vi "TAT_Planner_creator.vi"(8 "error in (no error)":errorcluster) -> (0 "error out":errorcluster)   [LabVIEW 2017]
uses:
  <vilib>/addons/database/Connection.llb/Conn ObjectReference.ctl
  b1939813-2d0c-4b6e-8ee7-2e1edd5edc28.vi
  <vilib>/Utility/config.llb/Read Key (I32).vi
  <vilib>/Utility/config.llb/Read Key (String).vi
  <userlib>/_OpenG.lib/array/array.llb/Remove Duplicates from 1D Array (String)__ogtk.vi
  <vilib>/Utility/config.llb/NI_LVConfig.lvlib
  <vilib>/addons/database/NI_Database_API.lvlib
panel:
  in  "BOX CALCULATION":bool
  out "PART LIST 6":string(tree)
  out "PART LIST 5":string(tree)
  out "PART LIST 4":string(tree)
  out "PART LIST 3":string(tree)
  out "PART LIST 2":string(tree)
  out "PART LIST 1":string(tree)
  out "PLANNED TABLE":string[][](table)
  in  "QTY 6":u32
  in  "TABLE DRAWING 6":string(combo)
  in  "COLOR 6":string(combo)
  in  "QTY 5":u32
  in  "TABLE DRAWING 5":string(combo)
  in  "COLOR 5":string(combo)
  in  "QTY 4":u32
  in  "TABLE DRAWING 4":string(combo)
  in  "COLOR 4":string(combo)
  in  "QTY 3":u32
  in  "TABLE DRAWING 3":string(combo)
  in  "COLOR 3":string(combo)
  in  "QTY 2":u32
  in  "TABLE DRAWING 2":string(combo)
  in  "COLOR 2":string(combo)
  in  "QTY 1":u32
  out "Array 2":string[][](array[string])
  out "Array":string[][](array[string])
  in  "TABLE DRAWING 1":string(combo)
  in  "WORK ORDER":string
  in  "COUNTRY":string(combo)
  in  "COLOR 1":string(combo)
  in  "MODEL":string(combo)
  in  "PLAN DATE":timestamp format="%<%x>T"
  in  "Cancle":bool
  in  "EDIT & SAVE":bool
  in  "CHILD PART CLUSTER":T1
  in  "CANCLE 3":bool
  in  "PRINTING":bool
  in  "Manual print":bool
  in  "Cancle 2":bool
  in  "Delete Button":bool
  in  "HOME":bool
  in  "UPDATE TABLE":bool
  in  "Tab Control":enum32{"Child Part Creator", "Varient Adding"}(tab)
  in  "CHILD PART NAME":string(combo)
  in  "Save Button":bool
  in  "QTY PER BOX":i32=1 min=1 max=100 step=1
  in  "Delete Square":bool
  in  "BOX WEIGHT":u16=1 min=1 max=100 step=1 format="%.0f gm"
  in  "BOX RH PART QUANTITY":u16=1 min=1 max=100 step=1
  in  "PART NUMBER":u16=1 min=1 max=100 step=1
  out "Varient Details":string[][](table)
  # "Export Plan Creator"
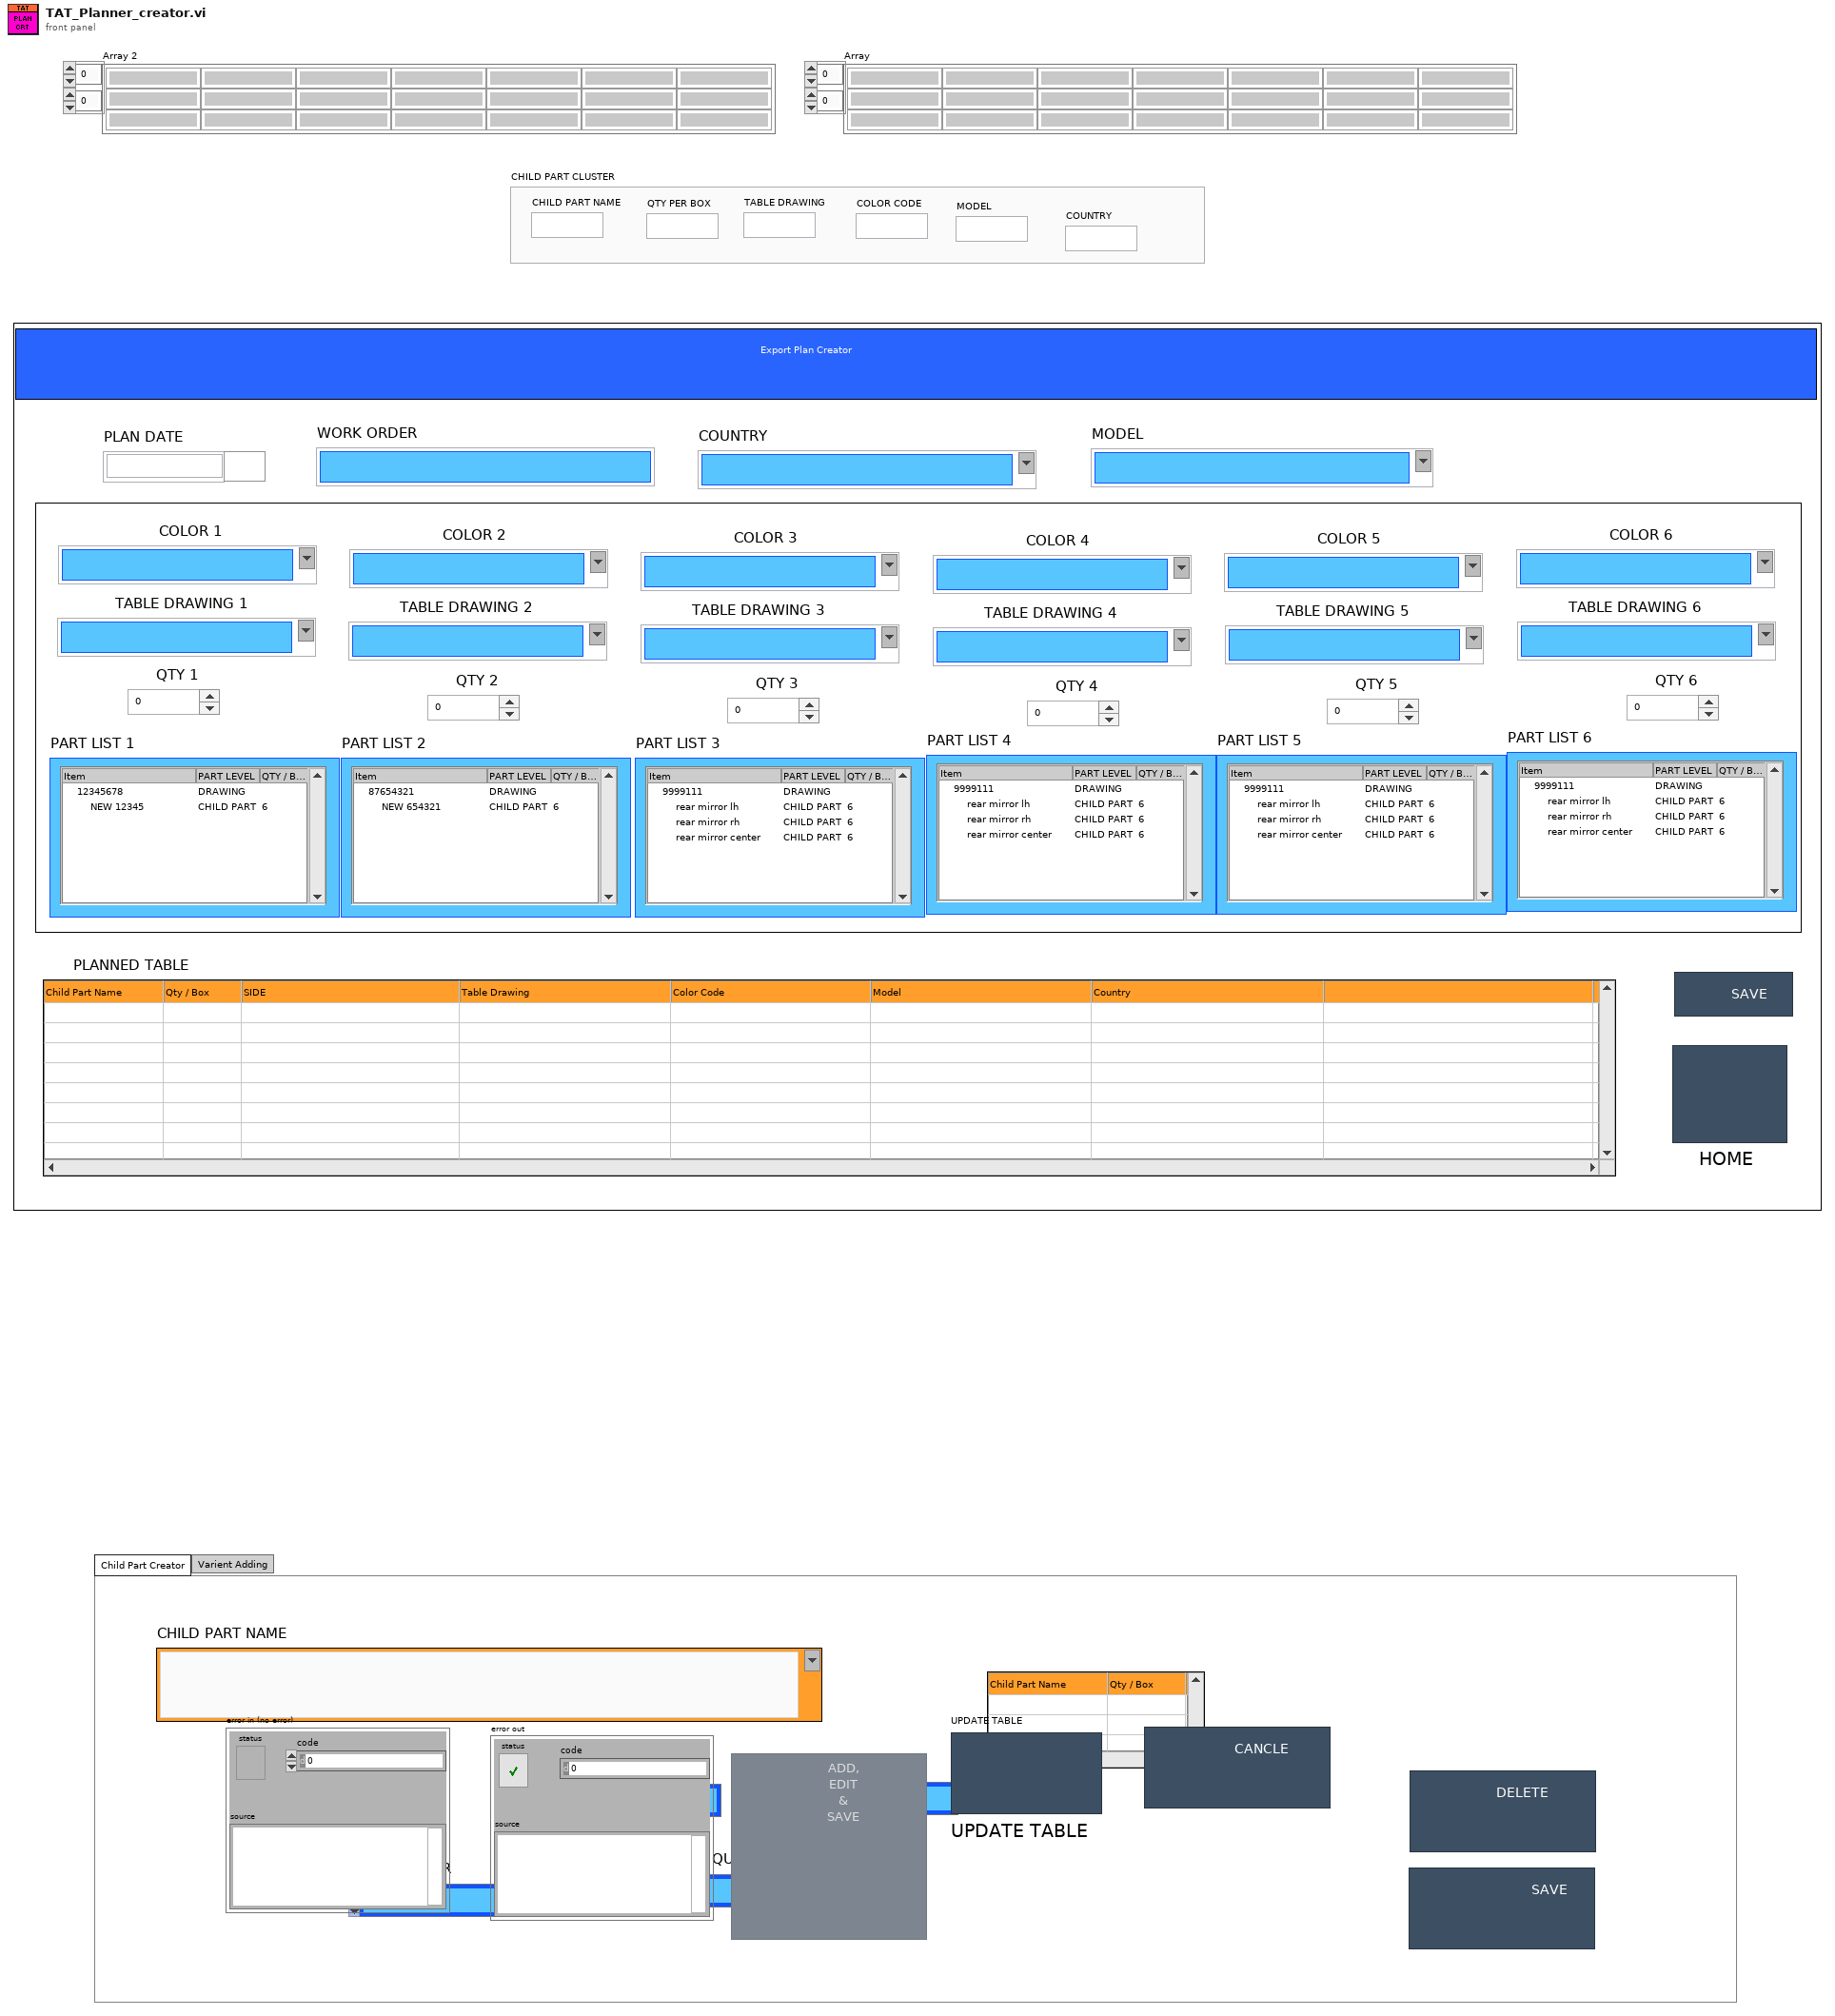
[diagram p1: front panel]
types:
  T1 = cluster{"CHILD PART NAME":string, "QTY PER BOX":string, "TABLE DRAWING":string, "COLOR CODE":string, "MODEL":string, "COUNTRY":string}
  T2 = enum32{"invalid app kind", "Development System", "Run Time System", "Student Edition", "Embedded LabVIEW", "Evaluation", "Custom"}
  T3 = typedef "NI_Database_API.lvlib/Conn ObjectReference.ctl" = refnum<k1>
  T4 = cluster{"Varient number":u16, "Part name":string, "connection reference":T3, "Batch_Size":u16, "PART_NO":string, "TORISHI_CODE":string, "scanner com":refnum<visa-resource-name>, "Part Name List":string[], "Varient path":path, "Current Varient path":path, "Communication path":path, "Package path":path, "Part PRN path":path, "Station2 printer IP":string, "Station1 printer IP":string, "Current Serial Number":string, "Station1_QR":string, "Serial_Number":path, "PRIVIOUS code":string[], "Barcode station2 log":string, "Barcode station2 Up":string, "HARNESS CODE":string, "Station 1 bypass":bool}
  T5 = cluster{"COLOR":string[], "MODEL":string[], "TABLE DRAWING":string[], "COUNTRY":string[]}
  T6 = typedef "NI_LVConfig.lvlib/Config Data RefNum.ctl" = refnum<k1>
  T7 = cluster{"QTY PER BOX":i32, "TABLE DRAWING":string, "COLOR CODE":string, "MODEL":string, "COUNTRY":string}
  T8 = enum8{"Enabled", "Disabled", "Disabled and Grayed Out"}
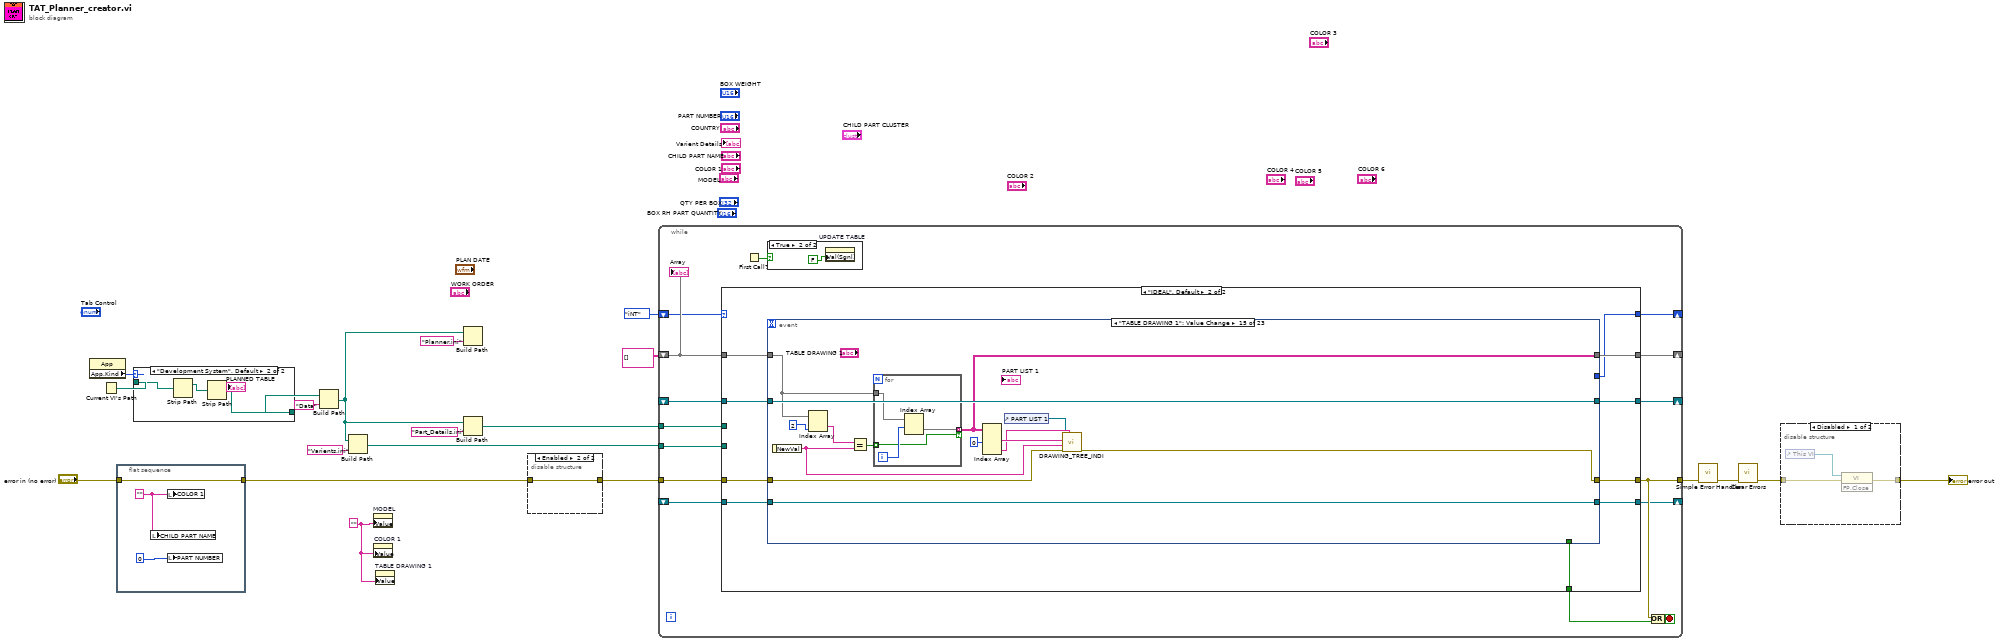
[diagram p0: block diagram]
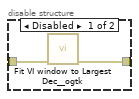
[diagram p2: hidden frame]
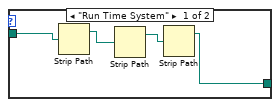
[diagram p4: hidden frame]
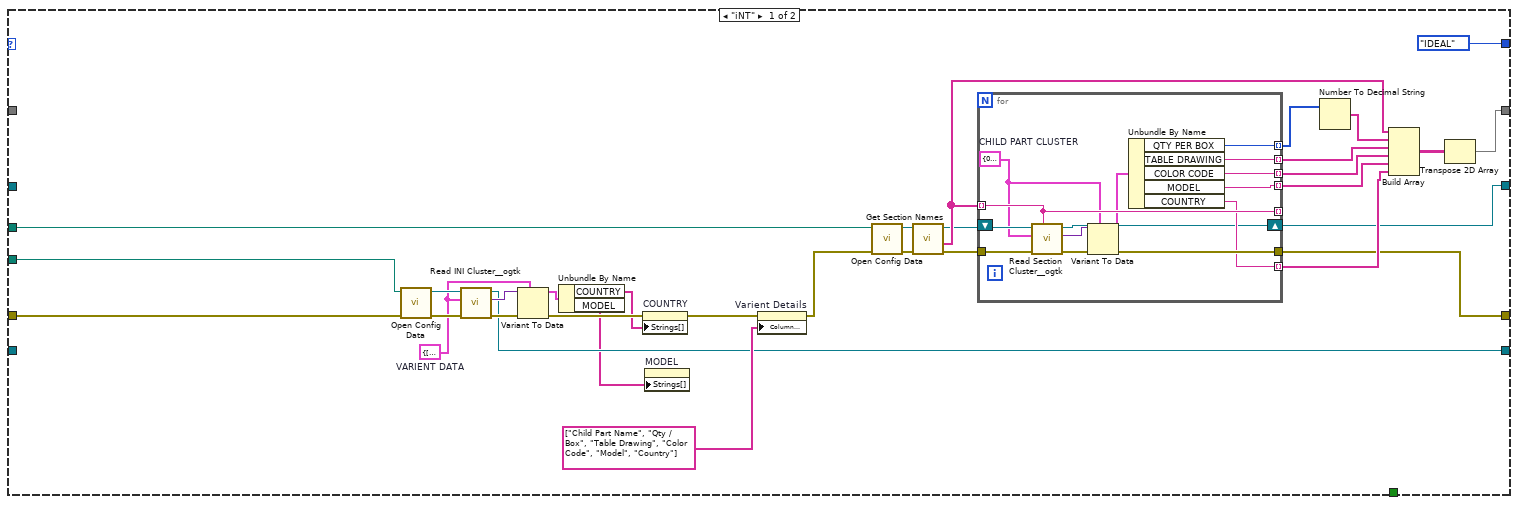
[diagram p5: hidden frame]
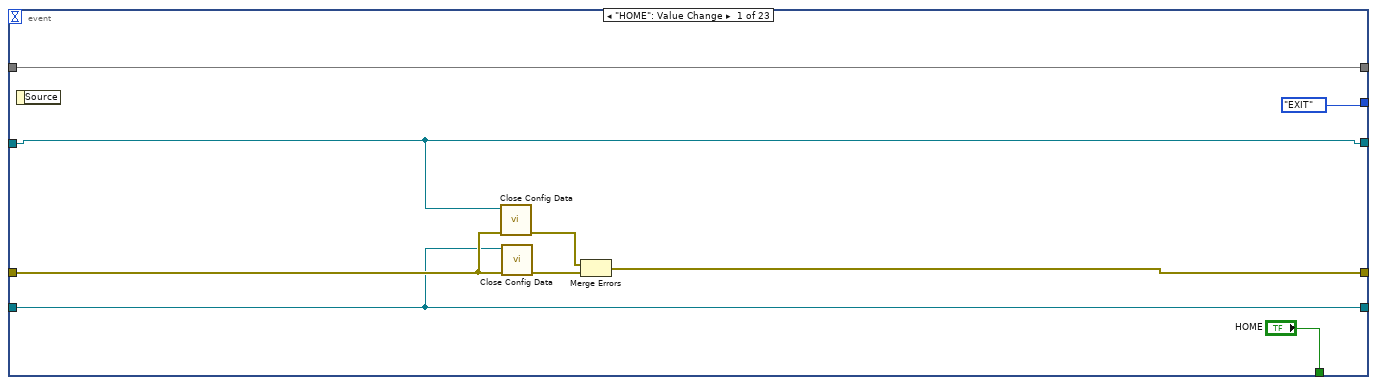
[diagram p6: hidden frame]
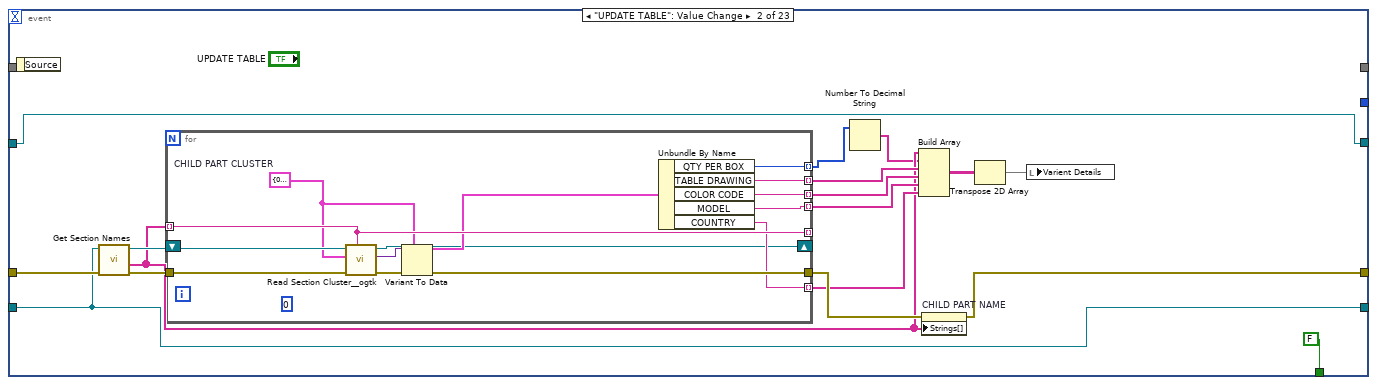
[diagram p7: hidden frame]
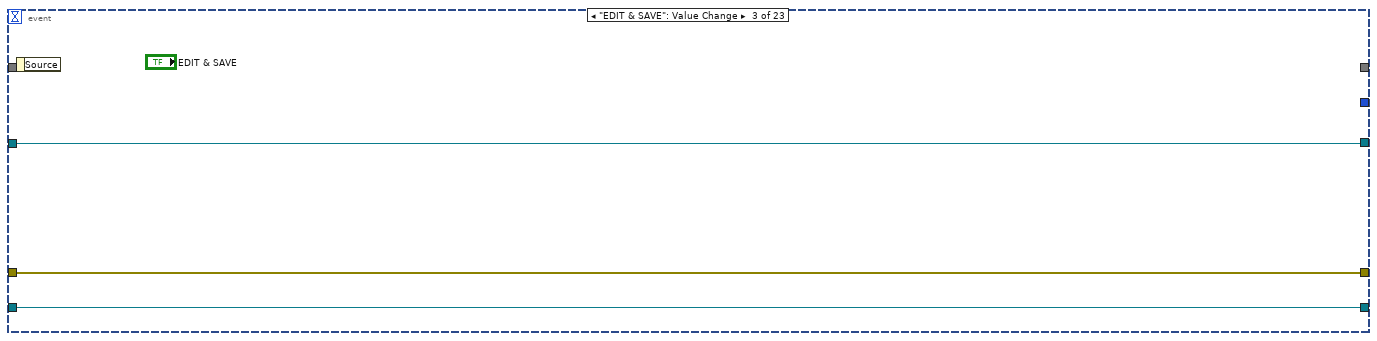
[diagram p8: hidden frame]
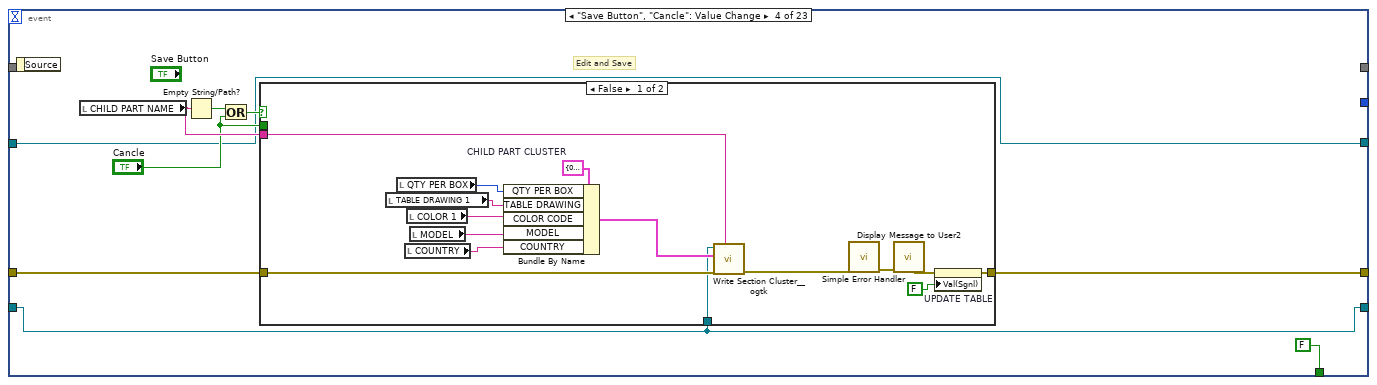
[diagram p9: hidden frame]
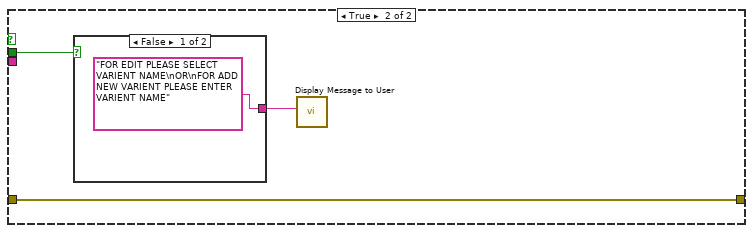
[diagram p10: hidden frame]
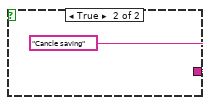
[diagram p11: hidden frame]
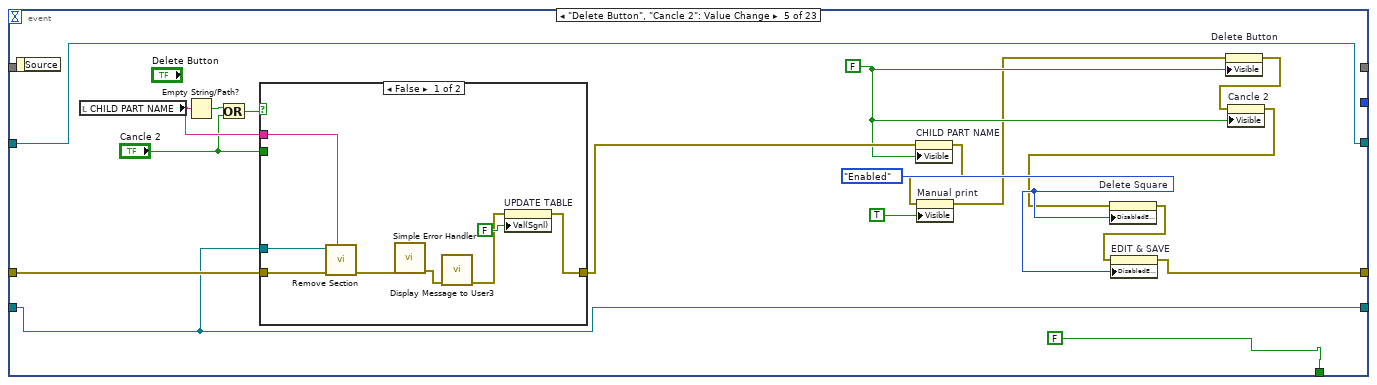
[diagram p12: hidden frame]
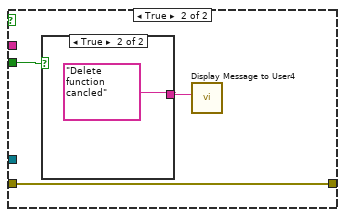
[diagram p13: hidden frame]
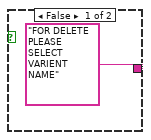
[diagram p14: hidden frame]
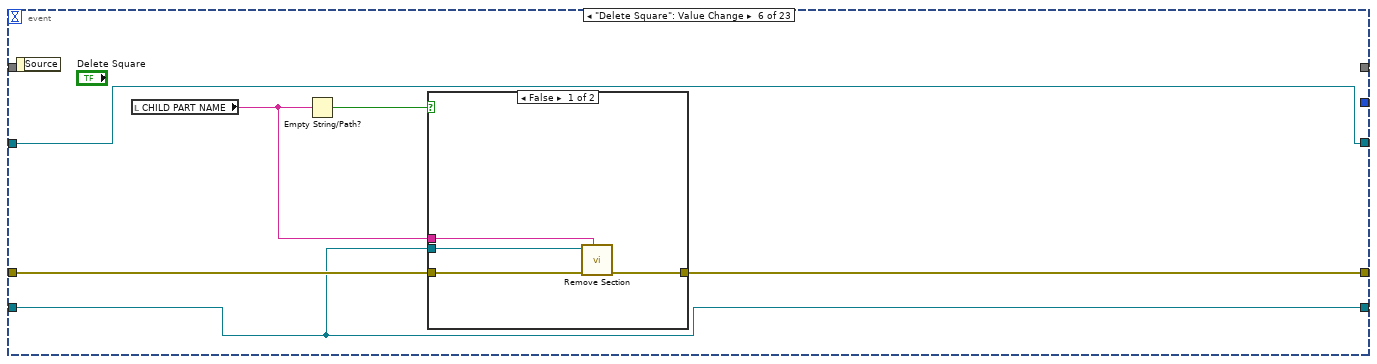
[diagram p15: hidden frame]
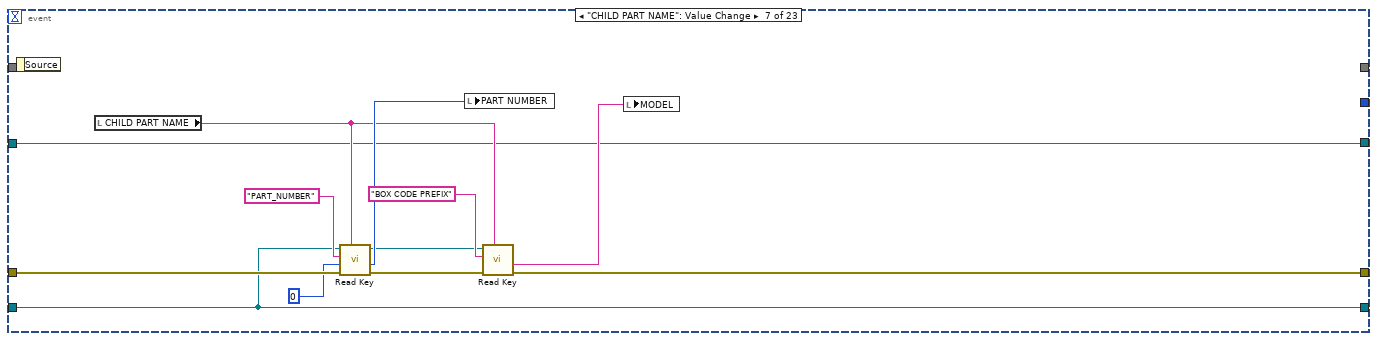
[diagram p17: hidden frame]
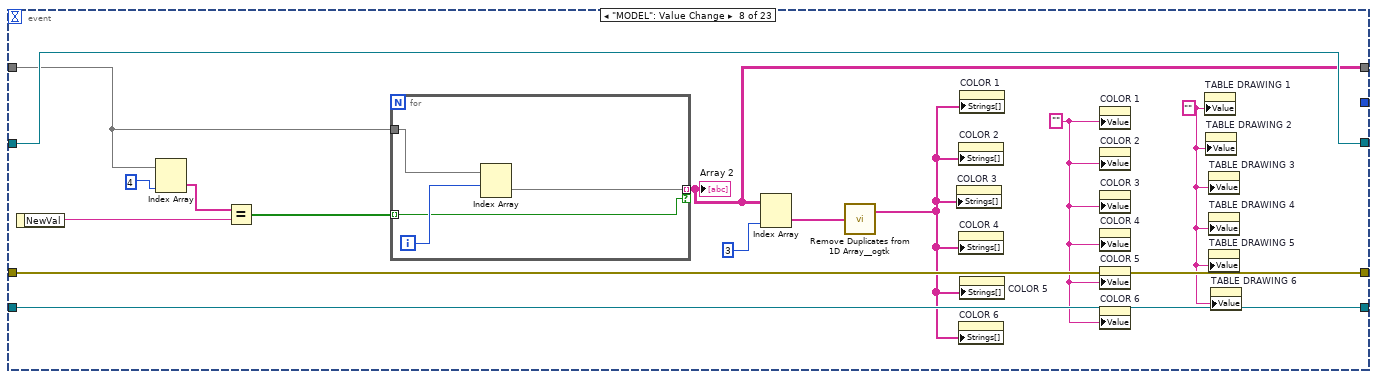
[diagram p18: hidden frame]
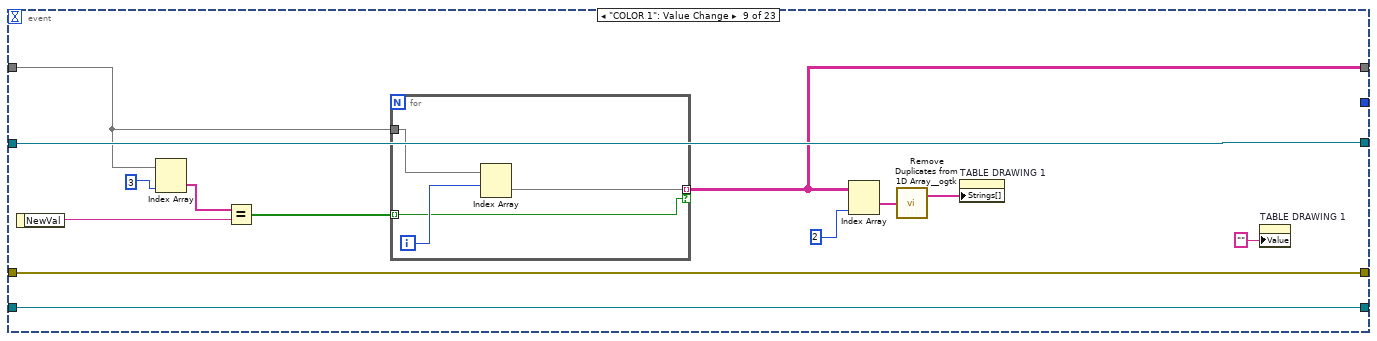
[diagram p19: hidden frame]
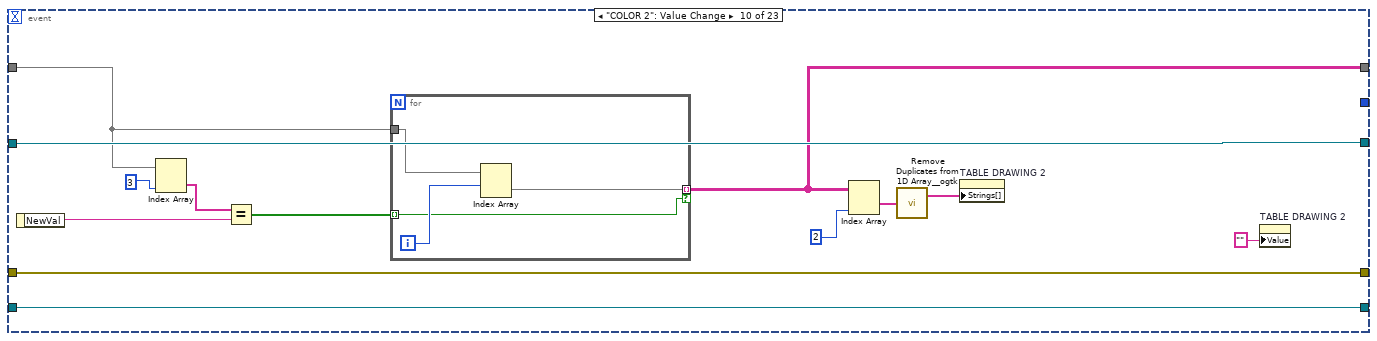
[diagram p20: hidden frame]
diagram:
  w4 = ""
  n1 = property class="App"() -> ("App.Kind"=w15:T2)  [unwired: 2 in, 2 out]
  n2 = Current VI's Path() -> (path=w16:path)
  n3 = flat-sequence {
    tunnel: [w21] -> w11
    tunnel: "error in (no error)" -> [w21]
    frame #0 {
      w23 = "" ("PART NUMBER")
      n4 = local write "CHILD PART NAME"(w23) -> ()
      n5 = local write "COLOR 1"(w23) -> ()
      n6 = local write "PART NUMBER"(u16 0 ("BATCH SIZE")) -> ()
    }
  }
  n7 = case shown="\"Development System\", Default" w15 {
    tunnel: w16 -> [w25 w29]
    tunnel: [w24 w28] -> w9
    frame "Run Time System" {
      n8 = Strip Path(path=w25) -> (stripped path=w27:path)  [unwired: 1 out]
      n9 = Strip Path(path=w27) -> (stripped path=w26:path)  [unwired: 1 out]
      n10 = Strip Path(path=w26) -> (stripped path=w24:path)  [unwired: 1 out]
    }
    frame "Development System", Default {
      n11 = Strip Path(path=w29) -> (stripped path=w30:path)  [unwired: 1 out]
      n12 = Strip Path(path=w30) -> (stripped path=w28:path)  [unwired: 1 out]
    }
  }
  n13 = Build Path(base path=w9, name or relative path="Data") -> (appended path=w6:path)
  n14 = Build Path(base path=w6, name or relative path="Varients.ini") -> (appended path=w2:path)
  n15 = property on="MODEL" class="CmbBox"("Value"=w4) -> ()  [unwired: 2 in, 2 out]
  n16 = property on="COLOR 1" class="CmbBox"("Value"=w4) -> ()  [unwired: 2 in, 2 out]
  n17 = property on="TABLE DRAWING 1" class="CmbBox"("Value"=w4) -> ()  [unwired: 2 in, 2 out]
  n18 = Build Path(base path=w6, name or relative path="Planner.ini") -> ()  [unwired: 1 out]
  n19 = Build Path(base path=w6, name or relative path="Part_Details.ini") -> (appended path=w7:path)
  n20 = disable-structure shown="Enabled" {
    disable-tunnel: w11 -> [w32 w33]
    disable-tunnel: [w31 w33] -> w8
    frame Disabled {
      n21 = call <userlib>:"Fit VI window to Largest Dec__ogtk.vi"("error in (no error)"=w32) -> ("error out"=w31:errorcluster)  [unwired: 5 in, 1 out]
    }
    frame Enabled {
    }
  }
  n22 = while {
    tunnel: w8 -> [w47]
    tunnel: [w45] -> w17
    tunnel: w7 -> [w40]
    shift-right: [w43] -> _
    shift-left: string[][] [] -> [w42]
    shift-right: [w34] -> _
    shift-left: enum16{"iNT", "IDEAL", "EXIT"}."iNT" -> [w41]
    shift-right: [w39] -> _
    shift-left: _ -> [w38]
    tunnel: w2 -> [w37]
    shift-right: [w36] -> _
    shift-left: _ -> [w35]
    stop <- w46 stop-if-true
    n23 = case shown="\"IDEAL\", Default" w41 {
      tunnel: [_ w104] -> w48
      tunnel: w47 -> [w54 w103]
      tunnel: [w70 w102] -> w45
      tunnel: [w65 w101] -> w43
      tunnel: w42 -> [_ w100]
      tunnel: w40 -> [w68 _]
      tunnel: [w66 w98] -> w39
      tunnel: w38 -> [_ w99]
      tunnel: w37 -> [w52 _]
      tunnel: [w51 w96] -> w36
      tunnel: w35 -> [_ w97]
      tunnel: [enum16{"iNT", "IDEAL", "EXIT"}."IDEAL" w95] -> w34
      frame "iNT" {
        w56 = T5 {"COLOR"=[], "MODEL"=[], "TABLE DRAWING"=[], "COUNTRY"=[]}  # VARIENT DATA
        n24 = call <vilib>:"Open Config Data.vi"("error in (no error)"=w54, "configuration file path"=w52) -> ("error out"=w62:errorcluster, "refnum"=w63:T6)  [unwired: 7 in, 1 out]
        n25 = call <userlib>:"Read INI Cluster__ogtk.vi"("error in (no error)"=w62, "INI Fomatted Cluster Type"=w56, "refnum"=w63) -> ("error out"=w61:errorcluster, "INI Fomatted Cluster"=w64:variant, "dup refnum"=w51:T6)  [unwired: 4 in, 2 out]
        n26 = Variant To Data(error in=w61, type=w56, Variant=w64) -> (data=w58:T5, error out=w60:errorcluster)
        n27 = Unbundle By Name(w58) -> ("COUNTRY"=w57:string[], "MODEL"=w49:string[])
        n28 = property on="COUNTRY" class="CmbBox"(error in=w60, "Strings[]"=w57) -> (error out=w59:errorcluster)  [unwired: 1 in, 1 out]
        n29 = property on="MODEL" class="CmbBox"("Strings[]"=w49) -> ()  [unwired: 2 in, 2 out]
        n30 = property on="Varient Details" class="Tbl (strict)"(error in=w59, "Column Headers[]"=string[] ["Child Part Name", "Qty / Box", "Table Drawing", "Color Code", "Model", "Country"] ("Column Header Strings[]")) -> (error out=w53:errorcluster)  [unwired: 1 in, 1 out]
        n31 = call <vilib>:"Open Config Data.vi"("error in (no error)"=w53, "configuration file path"=w68) -> ("error out"=w69:errorcluster, "refnum"=w67:T6)  [unwired: 7 in, 1 out]
        n32 = call <vilib>:"Get Section Names.vi"("error in (no error)"=w69, "refnum"=w67) -> ("error out"=w72:errorcluster, "section names"=w78:string[], "refnum out"=w73:T6)  [unwired: 7 in]
        n33 = for {
          tunnel: [w90] -> w70
          tunnel: w72 -> [w94]
          tunnel: w78 -> [w92] mode=indexing
          tunnel: [w92] -> _ mode=indexing
          tunnel: [w87] -> w79 mode=indexing
          tunnel: [w86] -> w74 mode=indexing
          tunnel: [w85] -> w75 mode=indexing
          tunnel: [w84] -> w76 mode=indexing
          tunnel: [w83] -> w77 mode=indexing
          shift-right: [w82] -> w66
          shift-left: w73 -> [w93]
          w81 = T7 {"QTY PER BOX"=0, "TABLE DRAWING"="", "COLOR CODE"="", "MODEL"="", "COUNTRY"=""}  # CHILD PART CLUSTER
          n34 = call <userlib>:"Read Section Cluster__ogtk.vi"("section (optional)"=w92, "error in (no error)"=w94, "Section Formatted Cluster Type"=w81, "refnum"=w93) -> ("error out"=w91:errorcluster, "Section Formatted Cluster"=w89:variant, "dup refnum"=w82:T6)  [unwired: 3 in, 2 out]
          n35 = Variant To Data(error in=w91, type=w81, Variant=w89) -> (data=w88:T7, error out=w90:errorcluster)
          n36 = Unbundle By Name(w88) -> ("QTY PER BOX"=w87:i32, "TABLE DRAWING"=w86:string, "COLOR CODE"=w85:string, "MODEL"=w84:string, "COUNTRY"=w83:string)
        }
        n37 = Number To Decimal String(number=w79) -> (decimal integer string=w80:string[])  [unwired: 1 in]
        n38 = Build Array(w78, w80, w74, w75, w76, w77) -> (w71:string[][])
        n39 = Transpose 2D Array(2D array=w71) -> (transposed array=w65:string[][])
      }
      frame "IDEAL", Default {
        n40 = event shown="[14] \"TABLE DRAWING 1\": Value Change" {
          selector: _ -> [_ _ _ _ _ _ _ _ _ _ _ _ _ _ _ _ _ _ _ _ _ _ _]
          dyn-events: _ -> [_ _ _ _ _ _ _ _ _ _ _ _ _ _ _ _ _ _ _ _ _ _ _]
          timeout: _ -> [_ _ _ _ _ _ _ _ _ _ _ _ _ _ _ _ _ _ _ _ _ _ _]
          tunnel: ["HOME" FALSE ("stop") _ FALSE ("stop") FALSE ("stop") _ _ _ _ _ _ _ _ _ _ _ _ _ _ _ _ _ _] -> w104
          tunnel: w103 -> [w111 w120 w147 w155 w193 w213 w230 w244 w261 w278 w295 w312 w329 w346 w364 w373 w387 w405 w423 w441 w459 w468 w485]
          tunnel: [w106 w119 w147 w150 w185 w212 w223 w244 w261 w278 w295 w312 w329 w346 w352 w373 w375 w393 w411 w429 w447 w467 w475] -> w102
          tunnel: [w110 _ _ _ _ _ _ w235 w251 w268 w285 w302 w319 w336 w357 w370 w380 w398 w416 w434 w452 _ _] -> w101
          tunnel: w100 -> [w110 _ _ _ _ _ _ w236 w252 w269 w286 w303 w320 w337 w358 w370 w381 w399 w417 w435 w453 _ _]
          tunnel: w99 -> [w109 w115 w146 w149 w178 w209 w220 w243 w259 w276 w293 w310 w327 w344 w363 w372 w386 w404 w422 w440 w458 w465 w472]
          tunnel: [w109 w115 w146 w149 w178 w209 w220 w243 w259 w276 w293 w310 w327 w344 w363 w372 w386 w404 w422 w440 w458 w465 w472] -> w98
          tunnel: w97 -> [w108 w114 w145 w148 w177 w208 w219 w242 w258 w275 w292 w309 w326 w343 w362 w371 w385 w403 w421 w439 w457 w464 w471]
          tunnel: [w108 w114 w145 w148 w177 w208 w219 w242 w258 w275 w292 w309 w326 w343 w362 w371 w385 w403 w421 w439 w457 w464 w471] -> w96
          tunnel: [enum16{"iNT", "IDEAL", "EXIT"}."EXIT" _ _ _ _ _ _ _ _ _ _ _ _ _ _ _ _ _ _ _ _ _ _] -> w95
          event "HOME": Value Change {
            n41 = event-data() -> ()  [unwired: 1 in, 1 out]
            n42 = call <vilib>:"Close Config Data.vi"("error in (no error)"=w111, "refnum"=w109) -> ("error out"=w105:errorcluster)  [unwired: 8 in, 1 out]
            n43 = call <vilib>:"Close Config Data.vi"("error in (no error)"=w111, "refnum"=w108) -> ("error out"=w112:errorcluster)  [unwired: 8 in, 1 out]
            n44 = Merge Errors(w105, w112) -> (w106:errorcluster)
          }
          event "UPDATE TABLE": Value Change {
            n45 = event-data() -> ()  [unwired: 1 in, 1 out]
            n46 = call <vilib>:"Get Section Names.vi"("error in (no error)"=w120, "refnum"=w114) -> ("error out"=w128:errorcluster, "section names"=w118:string[], "refnum out"=w127:T6)  [unwired: 7 in]
            n47 = for {
              tunnel: [w140] -> w126
              tunnel: w128 -> [w144]
              tunnel: w118 -> [w142] mode=indexing
              tunnel: [w142] -> _ mode=indexing
              tunnel: [w137] -> w117 mode=indexing
              tunnel: [w136] -> w124 mode=indexing
              tunnel: [w135] -> w123 mode=indexing
              tunnel: [w134] -> w122 mode=indexing
              tunnel: [w133] -> w121 mode=indexing
              shift-right: [w132] -> _
              shift-left: w127 -> [w143]
              w131 = T7 {"QTY PER BOX"=0, "TABLE DRAWING"="", "COLOR CODE"="", "MODEL"="", "COUNTRY"=""}  # CHILD PART CLUSTER
              (unwired) 0 ("default value")
              n48 = call <userlib>:"Read Section Cluster__ogtk.vi"("section (optional)"=w142, "error in (no error)"=w144, "Section Formatted Cluster Type"=w131, "refnum"=w143) -> ("error out"=w141:errorcluster, "Section Formatted Cluster"=w139:variant, "dup refnum"=w132:T6)  [unwired: 3 in, 2 out]
              n49 = Variant To Data(error in=w141, type=w131, Variant=w139) -> (data=w138:T7, error out=w140:errorcluster)
              n50 = Unbundle By Name(w138) -> ("QTY PER BOX"=w137:i32, "TABLE DRAWING"=w136:string, "COLOR CODE"=w135:string, "MODEL"=w134:string, "COUNTRY"=w133:string)
            }
            n51 = Number To Decimal String(number=w117) -> (decimal integer string=w116:string[])  [unwired: 1 in]
            n52 = Build Array(w118, w116, w124, w123, w122, w121) -> (w129:string[][])
            n53 = property on="CHILD PART NAME" class="CmbBox"(error in=w126, "Strings[]"=w118) -> (error out=w119:errorcluster)  [unwired: 1 in, 1 out]
            n54 = Transpose 2D Array(2D array=w129) -> (transposed array=w125:string[][])
            n55 = local write "Varient Details"(w125) -> ()
          }
          event "EDIT & SAVE": Value Change {
            n56 = event-data() -> ()  [unwired: 1 in, 1 out]
          }
          event "Save Button", "Cancle": Value Change {
            # "Edit and Save"
            n57 = event-data() -> ()  [unwired: 1 in, 1 out]
            n58 = local read "CHILD PART NAME"() -> (w154:string)
            n59 = Empty String/Path?(string/path=w154) -> (empty?=w153:bool)
            n60 = Or(x=w153, y="Cancle") -> (x .or. y?=w152:bool)
            n61 = case shown="False" w152 {
              tunnel: w155 -> [w171 w174]
              tunnel: [w169 w174] -> w150
              tunnel: w154 -> [w165 _]
              tunnel: "Cancle" -> [_ w172]
              tunnel: w148 -> [w157 _]
              frame False {
                w159 = T7 {"QTY PER BOX"=0, "TABLE DRAWING"="", "COLOR CODE"="", "MODEL"="", "COUNTRY"=""}  # CHILD PART CLUSTER
                n62 = local read "TABLE DRAWING 1"() -> (w161:string)
                n63 = local read "QTY PER BOX"() -> (w160:i32)
                n64 = local read "COUNTRY"() -> (w164:string)
                n65 = local read "COLOR 1"() -> (w162:string)
                n66 = local read "MODEL"() -> (w163:string)
                n67 = Bundle By Name(cluster=w159, "QTY PER BOX"=w160, "TABLE DRAWING"=w161, "COLOR CODE"=w162, "MODEL"=w163, "COUNTRY"=w164) -> (w158:T7)
                n68 = call <userlib>:"Write Section Cluster__ogtk.vi"("section (optional)"=w165, "error in (no error)"=w171, "Section Formatted Cluster"=w158, "refnum"=w157) -> ("error out"=w166:errorcluster)  [unwired: 6 in, 1 out]
                n69 = call <vilib>:"Simple Error Handler.vi"("error in (no error)"=w166) -> ("error out"=w168:errorcluster)  [unwired: 4 in, 4 out]
                n70 = call "Display Message to User2"("error in (no error)"=w168) -> ("error out"=w167:errorcluster)  [unwired: 9 in, 1 out]
                n71 = property on="UPDATE TABLE" class="Bool (strict)"(error in=w167, "Val(Sgnl)"=FALSE) -> (error out=w169:errorcluster)  [unwired: 1 in, 1 out]
              }
              frame True {
                n72 = case shown="False" w172 {
                  tunnel: ["FOR EDIT PLEASE SELECT VARIENT NAME\nOR\nFOR ADD NEW VARIENT PLEASE ENTER VARIENT NAME" "Cancle saving"] -> w173
                  frame False {
                  }
                  frame True {
                  }
                }
                n73 = call "Display Message to User"("Message"=w173) -> ()  [unwired: 9 in, 2 out]
              }
            }
          }
          event "Delete Button", "Cancle 2": Value Change {
            w187 = T8."Enabled" ("Disabled")
            w182 = FALSE
            n74 = event-data() -> ()  [unwired: 1 in, 1 out]
            n75 = local read "CHILD PART NAME"() -> (w192:string)
            n76 = Empty String/Path?(string/path=w192) -> (empty?=w191:bool)
            n77 = Or(x=w191, y="Cancle 2") -> (x .or. y?=w190:bool)
            n78 = case shown="False" w190 {
              tunnel: w193 -> [w197 w205]
              tunnel: [w201 w205] -> w186
              tunnel: w192 -> [w198 _]
              tunnel: "Cancle 2" -> [_ w204]
              tunnel: w177 -> [w195 _]
              frame False {
                n79 = call <vilib>:"Remove Section.vi"("section"=w198, "error in (no error)"=w197, "refnum"=w195) -> ("error out"=w196:errorcluster)  [unwired: 6 in, 2 out]
                n80 = call <vilib>:"Simple Error Handler.vi"("error in (no error)"=w196) -> ("error out"=w200:errorcluster)  [unwired: 4 in, 4 out]
                n81 = call "Display Message to User3"("error in (no error)"=w200) -> ("error out"=w199:errorcluster)  [unwired: 9 in, 1 out]
                n82 = property on="UPDATE TABLE" class="Bool (strict)"(error in=w199, "Val(Sgnl)"=FALSE) -> (error out=w201:errorcluster)  [unwired: 1 in, 1 out]
              }
              frame True {
                n83 = case shown="True" w204 {
                  tunnel: ["FOR DELETE PLEASE SELECT VARIENT NAME" "Delete function cancled"] -> w203
                  frame False {
                  }
                  frame True {
                  }
                }
                n84 = call "Display Message to User4"("Message"=w203) -> ()  [unwired: 9 in, 2 out]
              }
            }
            n85 = property on="CHILD PART NAME" class="CmbBox"(error in=w186, "Visible"=w182) -> (error out=w180:errorcluster)  [unwired: 1 in, 1 out]
            n86 = property on="Manual print" class="Bool"(error in=w180, "Visible"=TRUE) -> (error out=w179:errorcluster)  [unwired: 1 in, 1 out]
            n87 = property on="Delete Button" class="Bool"(error in=w179, "Visible"=w182) -> (error out=w184:errorcluster)  [unwired: 1 in, 1 out]
            n88 = property on="Cancle 2" class="Bool"(error in=w184, "Visible"=w182) -> (error out=w183:errorcluster)  [unwired: 1 in, 1 out]
            n89 = property on="Delete Square" class="Bool"(error in=w183, "DisabledEnum"=w187) -> (error out=w188:errorcluster)  [unwired: 1 in, 1 out]
            n90 = property on="EDIT & SAVE" class="Bool"(error in=w188, "DisabledEnum"=w187) -> (error out=w185:errorcluster)  [unwired: 1 in, 1 out]
          }
          event "Delete Square": Value Change {
            n91 = event-data() -> ()  [unwired: 1 in, 1 out]
            n92 = local read "CHILD PART NAME"() -> (w210:string)
            n93 = Empty String/Path?(string/path=w210) -> (empty?=w211:bool)
            n94 = case shown="False" w211 {
              tunnel: w213 -> [w217 w218]
              tunnel: [w216 w218] -> w212
              tunnel: w210 -> [w215 _]
              tunnel: w208 -> [w214 _]
              frame False {
                n95 = call <vilib>:"Remove Section.vi"("section"=w215, "error in (no error)"=w217, "refnum"=w214) -> ("error out"=w216:errorcluster)  [unwired: 6 in, 2 out]
              }
              frame True {
              }
            }
          }
          event "CHILD PART NAME": Value Change {
            n96 = event-data() -> ()  [unwired: 1 in, 1 out]
            n97 = local read "CHILD PART NAME"() -> (w222:string)
            n98 = call-poly <vilib>:"Read Key.vi"("section"=w222, "error in (no error)"=w230, "default value"=0, "key"="PART_NUMBER", "refnum"=w219) -> ("error out"=w226:errorcluster, "value"=w228:i32, "refnum out"=w224:T6)  [unwired: 3 in, 1 out]
            n99 = local write "PART NUMBER"(w228) -> ()
            n100 = call-poly <vilib>:"Read Key.vi"("section"=w222, "error in (no error)"=w226, "key"="BOX CODE PREFIX", "refnum"=w224) -> ("error out"=w223:errorcluster, "value"=w221:string)  [unwired: 4 in, 2 out]
            n101 = local write "MODEL"(w221) -> ()
          }
          event "MODEL": Value Change {
            w234 = ""
            w233 = ""
            n102 = event-data() -> ("NewVal"=w240:string)  [unwired: 1 in]
            n103 = Index Array(array=w236, index (col)=4) -> (element=w241:string[])  [unwired: 1 in]
            n104 = Equal?(x=w241, y=w240) -> (x = y?=w238:bool[])
            n105 = for {
              tunnel: w238 -> [w245] mode=indexing
              tunnel: w236 -> [w248]
              tunnel: [w246] -> w235 mode=indexing if=w245
              i -> [w247]
              n106 = Index Array(array=w248, index (row)=w247) -> (element=w246:string[])  [unwired: 1 in]
            }
            "Array 2" <- w235
            n107 = Index Array(array=w235, index (col)=3 ("disabled index (col)")) -> (element=w232:string[])  [unwired: 1 in]
            n108 = call-poly <userlib>:"Remove Duplicates from 1D Array__ogtk.vi"("Input Array"=w232) -> ("Output Array"=w231:string[])  [unwired: 1 out]
            n109 = property on="COLOR 3" class="CmbBox"("Strings[]"=w231) -> ()  [unwired: 2 in, 2 out]
            n110 = property on="COLOR 2" class="CmbBox"("Strings[]"=w231) -> ()  [unwired: 2 in, 2 out]
            n111 = property on="COLOR 4" class="CmbBox"("Strings[]"=w231) -> ()  [unwired: 2 in, 2 out]
            n112 = property on="COLOR 6" class="CmbBox"("Strings[]"=w231) -> ()  [unwired: 2 in, 2 out]
            n113 = property on="COLOR 1" class="CmbBox"("Strings[]"=w231) -> ()  [unwired: 2 in, 2 out]
            n114 = property on="COLOR 5" class="CmbBox"("Strings[]"=w231) -> ()  [unwired: 2 in, 2 out]
            n115 = property on="COLOR 1" class="CmbBox"("Value"=w234) -> ()  [unwired: 2 in, 2 out]
            n116 = property on="COLOR 2" class="CmbBox"("Value"=w234) -> ()  [unwired: 2 in, 2 out]
            n117 = property on="COLOR 3" class="CmbBox"("Value"=w234) -> ()  [unwired: 2 in, 2 out]
            n118 = property on="COLOR 4" class="CmbBox"("Value"=w234) -> ()  [unwired: 2 in, 2 out]
            n119 = property on="COLOR 5" class="CmbBox"("Value"=w234) -> ()  [unwired: 2 in, 2 out]
            n120 = property on="COLOR 6" class="CmbBox"("Value"=w234) -> ()  [unwired: 2 in, 2 out]
            n121 = property on="TABLE DRAWING 1" class="CmbBox"("Value"=w233) -> ()  [unwired: 2 in, 2 out]
            n122 = property on="TABLE DRAWING 2" class="CmbBox"("Value"=w233) -> ()  [unwired: 2 in, 2 out]
            n123 = property on="TABLE DRAWING 3" class="CmbBox"("Value"=w233) -> ()  [unwired: 2 in, 2 out]
            n124 = property on="TABLE DRAWING 4" class="CmbBox"("Value"=w233) -> ()  [unwired: 2 in, 2 out]
            n125 = property on="TABLE DRAWING 5" class="CmbBox"("Value"=w233) -> ()  [unwired: 2 in, 2 out]
            n126 = property on="TABLE DRAWING 6" class="CmbBox"("Value"=w233) -> ()  [unwired: 2 in, 2 out]
          }
          event "COLOR 1": Value Change {
            n127 = event-data() -> ("NewVal"=w256:string)  [unwired: 1 in]
            n128 = Index Array(array=w252, index (col)=3) -> (element=w257:string[])  [unwired: 1 in]
            n129 = Equal?(x=w257, y=w256) -> (x = y?=w254:bool[])
            n130 = for {
              tunnel: w254 -> [w262] mode=indexing
              tunnel: w252 -> [w265]
              tunnel: [w263] -> w251 mode=indexing if=w262
              i -> [w264]
              n131 = Index Array(array=w265, index (row)=w264) -> (element=w263:string[])  [unwired: 1 in]
            }
            n132 = Index Array(array=w251, index (col)=2 ("disabled index (col)")) -> (element=w250:string[])  [unwired: 1 in]
            n133 = call-poly <userlib>:"Remove Duplicates from 1D Array__ogtk.vi"("Input Array"=w250) -> ("Output Array"=w249:string[])  [unwired: 1 out]
            n134 = property on="TABLE DRAWING 1" class="CmbBox"("Strings[]"=w249) -> ()  [unwired: 2 in, 2 out]
            n135 = property on="TABLE DRAWING 1" class="CmbBox"("Value"="") -> ()  [unwired: 2 in, 2 out]
          }
          event "COLOR 2": Value Change {
            n136 = event-data() -> ("NewVal"=w273:string)  [unwired: 1 in]
            n137 = Index Array(array=w269, index (col)=3) -> (element=w274:string[])  [unwired: 1 in]
            n138 = Equal?(x=w274, y=w273) -> (x = y?=w271:bool[])
            n139 = for {
              tunnel: w271 -> [w279] mode=indexing
              tunnel: w269 -> [w282]
              tunnel: [w280] -> w268 mode=indexing if=w279
              i -> [w281]
              n140 = Index Array(array=w282, index (row)=w281) -> (element=w280:string[])  [unwired: 1 in]
            }
            n141 = Index Array(array=w268, index (col)=2 ("disabled index (col)")) -> (element=w267:string[])  [unwired: 1 in]
            n142 = call-poly <userlib>:"Remove Duplicates from 1D Array__ogtk.vi"("Input Array"=w267) -> ("Output Array"=w266:string[])  [unwired: 1 out]
            n143 = property on="TABLE DRAWING 2" class="CmbBox"("Strings[]"=w266) -> ()  [unwired: 2 in, 2 out]
            n144 = property on="TABLE DRAWING 2" class="CmbBox"("Value"="") -> ()  [unwired: 2 in, 2 out]
          }
          event "COLOR 3": Value Change {
            n145 = event-data() -> ("NewVal"=w290:string)  [unwired: 1 in]
            n146 = Index Array(array=w286, index (col)=3) -> (element=w291:string[])  [unwired: 1 in]
            n147 = Equal?(x=w291, y=w290) -> (x = y?=w288:bool[])
            n148 = for {
              tunnel: w288 -> [w296] mode=indexing
              tunnel: w286 -> [w299]
              tunnel: [w297] -> w285 mode=indexing if=w296
              i -> [w298]
              n149 = Index Array(array=w299, index (row)=w298) -> (element=w297:string[])  [unwired: 1 in]
            }
            n150 = Index Array(array=w285, index (col)=2 ("disabled index (col)")) -> (element=w284:string[])  [unwired: 1 in]
            n151 = call-poly <userlib>:"Remove Duplicates from 1D Array__ogtk.vi"("Input Array"=w284) -> ("Output Array"=w283:string[])  [unwired: 1 out]
            n152 = property on="TABLE DRAWING 3" class="CmbBox"("Strings[]"=w283) -> ()  [unwired: 2 in, 2 out]
            n153 = property on="TABLE DRAWING 3" class="CmbBox"("Value"="") -> ()  [unwired: 2 in, 2 out]
          }
          event "COLOR 4": Value Change {
            n154 = event-data() -> ("NewVal"=w307:string)  [unwired: 1 in]
            n155 = Index Array(array=w303, index (col)=3) -> (element=w308:string[])  [unwired: 1 in]
            n156 = Equal?(x=w308, y=w307) -> (x = y?=w305:bool[])
            n157 = for {
              tunnel: w305 -> [w313] mode=indexing
              tunnel: w303 -> [w316]
              tunnel: [w314] -> w302 mode=indexing if=w313
              i -> [w315]
              n158 = Index Array(array=w316, index (row)=w315) -> (element=w314:string[])  [unwired: 1 in]
            }
            n159 = Index Array(array=w302, index (col)=2 ("disabled index (col)")) -> (element=w301:string[])  [unwired: 1 in]
            n160 = call-poly <userlib>:"Remove Duplicates from 1D Array__ogtk.vi"("Input Array"=w301) -> ("Output Array"=w300:string[])  [unwired: 1 out]
            n161 = property on="TABLE DRAWING 4" class="CmbBox"("Strings[]"=w300) -> ()  [unwired: 2 in, 2 out]
            n162 = property on="TABLE DRAWING 4" class="CmbBox"("Value"="") -> ()  [unwired: 2 in, 2 out]
          }
          event "COLOR 5": Value Change {
            n163 = event-data() -> ("NewVal"=w324:string)  [unwired: 1 in]
            n164 = Index Array(array=w320, index (col)=3) -> (element=w325:string[])  [unwired: 1 in]
            n165 = Equal?(x=w325, y=w324) -> (x = y?=w322:bool[])
            n166 = for {
              tunnel: w322 -> [w330] mode=indexing
              tunnel: w320 -> [w333]
              tunnel: [w331] -> w319 mode=indexing if=w330
              i -> [w332]
              n167 = Index Array(array=w333, index (row)=w332) -> (element=w331:string[])  [unwired: 1 in]
            }
            n168 = Index Array(array=w319, index (col)=2 ("disabled index (col)")) -> (element=w318:string[])  [unwired: 1 in]
            n169 = call-poly <userlib>:"Remove Duplicates from 1D Array__ogtk.vi"("Input Array"=w318) -> ("Output Array"=w317:string[])  [unwired: 1 out]
            n170 = property on="TABLE DRAWING 5" class="CmbBox"("Strings[]"=w317) -> ()  [unwired: 2 in, 2 out]
            n171 = property on="TABLE DRAWING 5" class="CmbBox"("Value"="") -> ()  [unwired: 2 in, 2 out]
          }
          event "COLOR 6": Value Change {
            n172 = event-data() -> ("NewVal"=w341:string)  [unwired: 1 in]
            n173 = Index Array(array=w337, index (col)=3) -> (element=w342:string[])  [unwired: 1 in]
            n174 = Equal?(x=w342, y=w341) -> (x = y?=w339:bool[])
            n175 = for {
              tunnel: w339 -> [w347] mode=indexing
              tunnel: w337 -> [w350]
              tunnel: [w348] -> w336 mode=indexing if=w347
              i -> [w349]
              n176 = Index Array(array=w350, index (row)=w349) -> (element=w348:string[])  [unwired: 1 in]
            }
            n177 = Index Array(array=w336, index (col)=2 ("disabled index (col)")) -> (element=w335:string[])  [unwired: 1 in]
            n178 = call-poly <userlib>:"Remove Duplicates from 1D Array__ogtk.vi"("Input Array"=w335) -> ("Output Array"=w334:string[])  [unwired: 1 out]
            n179 = property on="TABLE DRAWING 6" class="CmbBox"("Strings[]"=w334) -> ()  [unwired: 2 in, 2 out]
            n180 = property on="TABLE DRAWING 6" class="CmbBox"("Value"="") -> ()  [unwired: 2 in, 2 out]
          }
          event "TABLE DRAWING 1": Value Change {
            n181 = event-data() -> ("NewVal"=w355:string)  [unwired: 1 in]
            n182 = Index Array(array=w358, index (col)=2) -> (element=w361:string[])  [unwired: 1 in]
            n183 = Equal?(x=w361, y=w355) -> (x = y?=w359:bool[])
            n184 = for {
              tunnel: w359 -> [w365] mode=indexing
              tunnel: w358 -> [w368]
              tunnel: [w366] -> w357 mode=indexing if=w365
              i -> [w367]
              n185 = Index Array(array=w368, index (row)=w367) -> (element=w366:string[])  [unwired: 1 in]
            }
            n186 = Index Array(array=w357, index (col) #1=0 ("disabled index (col)")) -> (element #1=w354:string[], element #2=w353:string[])  [unwired: 3 in]
            n187 = control-ref of="PART LIST 1"() -> (w351:refnum<vi>)
            n188 = call "DRAWING_TREE_INDI.vi"("Array"=w353, "error in (no error)"=w364, "NewVal"=w355, "Array 2"=w354, "TreeControl in"=w351) -> ("error out"=w352:errorcluster)  [unwired: 6 in]
          }
          event "BOX CALCULATION": Value Change {
            n189 = event-data() -> ()  [unwired: 1 in, 1 out]
            n190 = case shown="1, Default" "QTY 1" {
              frame 0 {
              }
              frame 1, Default {
              }
            }
          }
          event "TABLE DRAWING 2": Value Change {
            n191 = event-data() -> ("NewVal"=w378:string)  [unwired: 1 in]
            n192 = Index Array(array=w381, index (col)=2) -> (element=w384:string[])  [unwired: 1 in]
            n193 = Equal?(x=w384, y=w378) -> (x = y?=w382:bool[])
            n194 = for {
              tunnel: w382 -> [w388] mode=indexing
              tunnel: w381 -> [w391]
              tunnel: [w389] -> w380 mode=indexing if=w388
              i -> [w390]
              n195 = Index Array(array=w391, index (row)=w390) -> (element=w389:string[])  [unwired: 1 in]
            }
            n196 = Index Array(array=w380, index (col) #1=0 ("disabled index (col)")) -> (element #1=w377:string[], element #2=w376:string[])  [unwired: 3 in]
            n197 = control-ref of="PART LIST 2"() -> (w374:refnum<vi>)
            n198 = call "DRAWING_TREE_INDI.vi"("Array"=w376, "error in (no error)"=w387, "NewVal"=w378, "Array 2"=w377, "TreeControl in"=w374) -> ("error out"=w375:errorcluster)  [unwired: 6 in]
          }
          event "TABLE DRAWING 3": Value Change {
            n199 = event-data() -> ("NewVal"=w396:string)  [unwired: 1 in]
            n200 = Index Array(array=w399, index (col)=2) -> (element=w402:string[])  [unwired: 1 in]
            n201 = Equal?(x=w402, y=w396) -> (x = y?=w400:bool[])
            n202 = for {
              tunnel: w400 -> [w406] mode=indexing
              tunnel: w399 -> [w409]
              tunnel: [w407] -> w398 mode=indexing if=w406
              i -> [w408]
              n203 = Index Array(array=w409, index (row)=w408) -> (element=w407:string[])  [unwired: 1 in]
            }
            n204 = Index Array(array=w398, index (col) #1=0 ("disabled index (col)")) -> (element #1=w395:string[], element #2=w394:string[])  [unwired: 3 in]
            n205 = control-ref of="PART LIST 3"() -> (w392:refnum<vi>)
            n206 = call "DRAWING_TREE_INDI.vi"("Array"=w394, "error in (no error)"=w405, "NewVal"=w396, "Array 2"=w395, "TreeControl in"=w392) -> ("error out"=w393:errorcluster)  [unwired: 6 in]
          }
          event "TABLE DRAWING 4": Value Change {
            n207 = event-data() -> ("NewVal"=w414:string)  [unwired: 1 in]
            n208 = Index Array(array=w417, index (col)=2) -> (element=w420:string[])  [unwired: 1 in]
            n209 = Equal?(x=w420, y=w414) -> (x = y?=w418:bool[])
            n210 = for {
              tunnel: w418 -> [w424] mode=indexing
              tunnel: w417 -> [w427]
              tunnel: [w425] -> w416 mode=indexing if=w424
              i -> [w426]
              n211 = Index Array(array=w427, index (row)=w426) -> (element=w425:string[])  [unwired: 1 in]
            }
            n212 = Index Array(array=w416, index (col) #1=0 ("disabled index (col)")) -> (element #1=w413:string[], element #2=w412:string[])  [unwired: 3 in]
            n213 = control-ref of="PART LIST 4"() -> (w410:refnum<vi>)
            n214 = call "DRAWING_TREE_INDI.vi"("Array"=w412, "error in (no error)"=w423, "NewVal"=w414, "Array 2"=w413, "TreeControl in"=w410) -> ("error out"=w411:errorcluster)  [unwired: 6 in]
          }
          event "TABLE DRAWING 5": Value Change {
            n215 = event-data() -> ("NewVal"=w432:string)  [unwired: 1 in]
            n216 = Index Array(array=w435, index (col)=2) -> (element=w438:string[])  [unwired: 1 in]
            n217 = Equal?(x=w438, y=w432) -> (x = y?=w436:bool[])
            n218 = for {
              tunnel: w436 -> [w442] mode=indexing
              tunnel: w435 -> [w445]
              tunnel: [w443] -> w434 mode=indexing if=w442
              i -> [w444]
              n219 = Index Array(array=w445, index (row)=w444) -> (element=w443:string[])  [unwired: 1 in]
            }
            n220 = Index Array(array=w434, index (col) #1=0 ("disabled index (col)")) -> (element #1=w431:string[], element #2=w430:string[])  [unwired: 3 in]
            n221 = control-ref of="PART LIST 5"() -> (w428:refnum<vi>)
            n222 = call "DRAWING_TREE_INDI.vi"("Array"=w430, "error in (no error)"=w441, "NewVal"=w432, "Array 2"=w431, "TreeControl in"=w428) -> ("error out"=w429:errorcluster)  [unwired: 6 in]
          }
          event "TABLE DRAWING 6": Value Change {
            n223 = event-data() -> ("NewVal"=w450:string)  [unwired: 1 in]
            n224 = Index Array(array=w453, index (col)=2) -> (element=w456:string[])  [unwired: 1 in]
            n225 = Equal?(x=w456, y=w450) -> (x = y?=w454:bool[])
            n226 = for {
              tunnel: w454 -> [w460] mode=indexing
              tunnel: w453 -> [w463]
              tunnel: [w461] -> w452 mode=indexing if=w460
              i -> [w462]
              n227 = Index Array(array=w463, index (row)=w462) -> (element=w461:string[])  [unwired: 1 in]
            }
            n228 = Index Array(array=w452, index (col) #1=0 ("disabled index (col)")) -> (element #1=w449:string[], element #2=w448:string[])  [unwired: 3 in]
            n229 = control-ref of="PART LIST 6"() -> (w446:refnum<vi>)
            n230 = call "DRAWING_TREE_INDI.vi"("Array"=w448, "error in (no error)"=w459, "NewVal"=w450, "Array 2"=w449, "TreeControl in"=w446) -> ("error out"=w447:errorcluster)  [unwired: 6 in]
          }
          event "Manual print": Value Change {
            w466 = TRUE
            n231 = event-data() -> ()  [unwired: 1 in, 1 out]
            n232 = property on="CHILD PART NAME" class="CmbBox"(error in=w468, "Visible"=w466) -> (error out=w470:errorcluster)  [unwired: 1 in, 1 out]
            n233 = property on="CANCLE 3" class="Bool"(error in=w470, "Visible"=w466) -> (error out=w469:errorcluster)  [unwired: 1 in, 1 out]
            n234 = property on="PRINTING" class="Bool"(error in=w469, "Visible"=w466) -> (error out=w467:errorcluster)  [unwired: 1 in, 1 out]
          }
          event "PRINTING", "CANCLE 3": Value Change {
            w476 = T8."Enabled" ("Disabled")
            w477 = FALSE
            n235 = event-data() -> ()  [unwired: 1 in, 1 out]
            n236 = local read "CHILD PART NAME"() -> (w482:string)
            n237 = Empty String/Path?(string/path=w482) -> (empty?=w484:bool)
            n238 = Or(x=w484, y="CANCLE 3") -> (x .or. y?=w483:bool)
            n239 = case shown="False" w483 {
              tunnel: w485 -> [w500 w512]
              tunnel: [w492 w512] -> w474
              tunnel: w482 -> [w488 _]
              tunnel: "CANCLE 3" -> [_ w510]
              tunnel: w471 -> [w486 _]
              frame False {
                n240 = call-poly <vilib>:"Read Key.vi"("section"=w488, "error in (no error)"=w500, "default value"=0, "key"="BATCH_SIZE", "refnum"=w486) -> ("error out"=w509:errorcluster, "value"=w491:i32, "refnum out"=w508:T6)  [unwired: 3 in, 1 out]
                n241 = call-poly <vilib>:"Read Key.vi"("section"=w488, "error in (no error)"=w509, "default value"=0, "key"="VARIENT_NO", "refnum"=w508) -> ("error out"=w506:errorcluster, "refnum out"=w505:T6)  [unwired: 3 in, 2 out]
                n242 = call-poly <vilib>:"Read Key.vi"("section"=w488, "error in (no error)"=w506, "key"="PART_NO", "refnum"=w505) -> ("error out"=w507:errorcluster, "value"=w489:string)  [unwired: 4 in, 2 out]
                n243 = Bundle By Name(cluster=T4 {"Varient number"=0, "Part name"="", "connection reference"=refnum, "Batch_Size"=0, "PART_NO"="", "TORISHI_CODE"="", "scanner com"="", "Part Name List"=[], "Varient path"=path "", "Current Varient path"=path "", "Communication path"=path "", "Package path"=path "", "Part PRN path"=path "", "Station2 printer IP"="", "Station1 printer IP"="", "Current Serial Number"="", "Station1_QR"="", "Serial_Number"=path "", "PRIVIOUS code"=[], "Barcode station2 log"="", "Barcode station2 Up"="", "HARNESS CODE"="", "Station 1 bypass"=FALSE} ("Cluster 2"), "Part name"=w488, "PART_NO"=w489, "TORISHI_CODE"=w488, "Batch_Size"=w491, "HARNESS CODE"=w488) -> ()  [unwired: 1 out]
                n244 = TCP Open Connection(remote port or service name=u16 6101, error in (no error)=w507) -> (connection ID=w497:refnum<k5>, error out=w496:errorcluster)  [unwired: 3 in]
                n245 = TCP Write(connection ID=w497, error in (no error)=w496) -> (connection ID out=w499:refnum<k5>, error out=w495:errorcluster)  [unwired: 2 in, 1 out]
                n246 = call "Stall Data Flow.vim"("value in"=w495, "milliseconds to wait"=u32 1000) -> ("value out"=w498:errorcluster)  [unwired: 1 out]
                n247 = TCP Close Connection(connection ID=w499, error in (no error)=w498) -> (error out=w492:errorcluster)  [unwired: 1 in, 1 out]
              }
              frame True {
                n248 = case shown="False" w510 {
                  tunnel: ["FOR PRINT SELECT VARIENT NAME." "Cancle saving"] -> w511
                  frame False {
                  }
                  frame True {
                  }
                }
                n249 = call "Display Message to User5"("Message"=w511) -> ()  [unwired: 9 in, 2 out]
              }
            }
            n250 = property on="CHILD PART NAME" class="CmbBox"(error in=w474, "Visible"=w477) -> (error out=w481:errorcluster)  [unwired: 1 in, 1 out]
            n251 = property on="PRINTING" class="Bool"(error in=w481, "Visible"=w477) -> (error out=w479:errorcluster)  [unwired: 1 in, 1 out]
            n252 = property on="CANCLE 3" class="Bool"(error in=w479, "Visible"=w477) -> (error out=w478:errorcluster)  [unwired: 1 in, 1 out]
            n253 = property on="Delete Square" class="Bool"(error in=w478, "DisabledEnum"=w476) -> (error out=w480:errorcluster)  [unwired: 1 in, 1 out]
            n254 = property on="EDIT & SAVE" class="Bool"(error in=w480, "DisabledEnum"=w476) -> (error out=w475:errorcluster)  [unwired: 1 in, 1 out]
          }
        }
      }
    }
    n255 = First Call?() -> (First Call?: T/F=w44:bool)
    n256 = case shown="True" w44 {
      frame False {
      }
      frame True {
        n257 = property on="UPDATE TABLE" class="Bool (strict)"("Val(Sgnl)"=FALSE) -> ()  [unwired: 2 in, 2 out]
      }
    }
    n258 = Or(x=w45, y=w48) -> (x .or. y?=w46:bool)
    "Array" <- w42
  }
  n259 = call <vilib>:"Simple Error Handler.vi"("error in (no error)"=w17) -> ("error out"=w20:errorcluster)  [unwired: 4 in, 4 out]
  n260 = call <vilib>:"Clear Errors.vi"("error in (no error)"=w20) -> ("error out"=w19:errorcluster)  [unwired: 5 in, 1 out]
  n261 = disable-structure shown="Disabled" {
    disable-tunnel: w19 -> [w518 w519]
    disable-tunnel: [w517 w519] -> w18
    frame Disabled {
      n262 = control-ref of="This VI"() -> (w516:refnum<vi>)
      n263 = invoke class="VI" method="FP.Close"(reference=w516, error in=w518) -> (error out=w517:errorcluster)  [unwired: 1 in, 2 out]
    }
    frame Enabled {
    }
  }
  "error out" <- w18
